vi "Variant Array to Spreadsheet__ogtk.vi"(7 "delimiter (Tab)":string="\t", 8 "2D Variant Array":variant[][](array[variant]), 10 "error in (no error)":errorcluster) -> (0 "spreadsheet string":string, 2 "error out":errorcluster)   [LabVIEW 2014]
doc: "Overcomes a limitation of \"Array to Spreadsheet String\" by allowing variant data types to be used. This VI supports variant data for all LabVIEW data types supported by \"Format Into String\". The \"format string\" for each Varriant element of the input array must be passed within each variant element as a variant attribute named \"Format String\"."
panel:
  # "[OpenG VI Tags] ***Do Not Remove***"
  # "Variant Array to Spreadsheet String.vi\n\nOvercomes a limitation of \"Array to Spreadsheet String\" by allowing variant data types to be used.\nThis VI supports variant data for all LabVIEW data types supported by \"Format Into String\".  The \"format string\" for each Varriant element of\nthe input array must be passed within each variant element as a variant attribute named \"Format String\".\n\nPlease visit http://www.OpenG.org to learn about the\nOpen Source LabVIEW software movement.\n\nNOTICE -- YOU MUST LEAVE THIS NOTICE IN PLACE.  PER THE TERMS OF THE LICENSE BELOW, YOU MAY SUBLICENSE THIS SOFTWARE \nIN ANY WAY THAT DOES NOT CONFLICT WITH THIS LICENSE.\n\n### BSD License (http://www.opensource.org/licenses/bsd-license.php) Begin ###\n \nCopyright (c) 2002, Jim Kring <jim@jimkring.com>\n\nAll rights reserved.\n\nRedistribution and use in source and binary forms, with or without modification, are permitted provided that the following conditions are met:\n\n    * Redistributions of source code must retain the above copyright notice, this list of conditions and the following disclaimer.\n    * Redistributions in binary form must reproduce the above copyright notice, this list of conditions and the following disclaimer in the \n       documentation and/or other materials provided with the distribution.\n    * Neither the name of SciWare, James Kring, Inc., nor the names of its contributors may be used to endorse or promote products derived \n       from this software without specific prior written permission.\n\nTHIS SOFTWARE IS PROVIDED BY THE COPYRIGHT HOLDERS AND CONTRIBUTORS \"AS IS\" AND ANY EXPRESS OR IMPLIED WARRANTIES, \nINCLUDING, BUT NOT LIMITED TO, THE IMPLIED WARRANTIES OF MERCHANTABILITY AND FITNESS FOR A PARTICULAR PURPOSE ARE \nDISCLAIMED. IN NO EVENT SHALL THE COPYRIGHT OWNER OR CONTRIBUTORS BE LIABLE FOR ANY DIRECT, INDIRECT, INCIDENTAL,\n SPECIAL, EXEMPLARY, OR CONSEQUENTIAL DAMAGES (INCLUDING, BUT NOT LIMITED TO, PROCUREMENT OF SUBSTITUTE GOODS OR \nSERVICES; LOSS OF USE, DATA, OR PROFITS; OR BUSINESS INTERRUPTION) HOWEVER CAUSED AND ON ANY THEORY OF LIABILITY, \nWHETHER IN CONTRACT, STRICT LIABILITY, OR TORT (INCLUDING NEGLIGENCE OR OTHERWISE) ARISING IN ANY WAY OUT OF THE USE \nOF THIS SOFTWARE, EVEN IF ADVISED OF THE POSSIBILITY OF SUCH DAMAGE.\n\n### BSD License End ###"
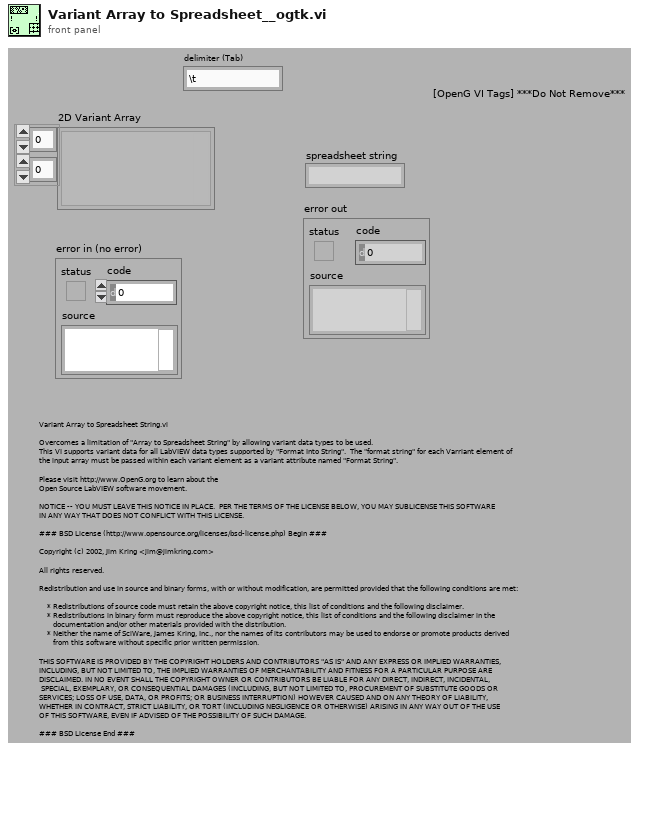
[diagram p1: front panel]
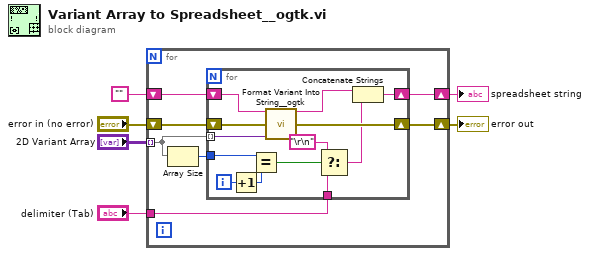
[diagram p0: block diagram]
diagram:
  n1 = for {
    tunnel: "2D Variant Array" -> [w10] mode=indexing
    shift-right: [w8] -> w1
    shift-left: "" -> [w13]
    tunnel: "delimiter (Tab)" -> [w9]
    shift-right: [w12] -> w2
    shift-left: "error in (no error)" -> [w7]
    n2 = Array Size(array=w10) -> (size(s)=w11:i32)
    n3 = for {
      tunnel: w10 -> [w26] mode=indexing
      shift-right: [w15] -> w8
      shift-left: w13 -> [w25]
      shift-right: [w23] -> w12
      shift-left: w7 -> [w24]
      tunnel: w11 -> [w21]
      tunnel: w9 -> [w17]
      i -> [w22]
      n4 = Increment(x=w22) -> (x+1=w20:i32)
      n5 = Equal?(x=w21, y=w20) -> (x = y?=w19:bool)
      n6 = call <userlib>:"Format Variant Into String__ogtk.vi"("Input String"=w25, "error in (no error)"=w24, "Variant"=w26) -> ("Output String"=w16:string, "error out"=w23:errorcluster)  [unwired: 11 in]
      n7 = Select(t="\r\n", s=w19, f=w17) -> (s? t:f=w14:string)
      n8 = Concatenate Strings(w16, w14) -> (w15:string)
    }
  }
  "error out" <- w2
  "spreadsheet string" <- w1
